vi "t1.vi"() -> ()   [LabVIEW 2017]
panel:
  in  "布尔 2":bool
  in  "布尔":bool
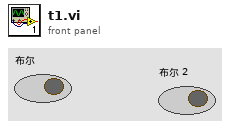
[diagram p1: front panel]
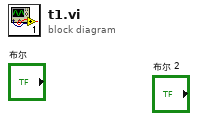
[diagram p0: block diagram]
diagram:
